vi "GPIB write expt GPIB.vi"(0 "Command list 1":T1(array[cluster]) {"Module" items=["TTL high                                                                                 ", "TTL low                          ", "Camera Strobe                   ", "CMOT", "Defaults                           ", "Fluorescence pulse           ", "IP trap                         ", "Kinetics OD image          ", "Kinetics picture", "Kinetics probe pulse", "MOT light only                ", "MOT off                                   ", "MOT on                         ", "Move cart                      ", "OD image                     ", "Optical pumping          ", "Picture                             ", "Probe Pulse", "Quadrupole trap             ", "IP off", "Utility Module 02           ", "Utility Module 03           ", "Molasses          ", "Utility Module 04     ", "Utility Module 05     ", "Utility Module 06     ", "Utility Module 07     ", "Utility Module 08     ", "Utility Module 09     ", "Utility Module 10     ", "Static DAC", "GPIB"]; "Abs Start Time" format="%.3f"}, 1 "End time":dbl=83073.546, 2 "Abs start time":dbl=62269.999980926514, 3 "do it!":bool=TRUE) -> ()   [LabVIEW 2017]
doc: "This sends out GPIB commands during the experiment (after the DIO (TTL) board has been triggered."
uses:
  globals/Modules global.vi
panel:
  out "Array 2":dbl[](array[numeric])
  out "Array":string[](array[string])
  out "sorted array":T1(array[cluster])
  out "total time":dbl
  out "start time":dbl=3231522488.434
  in  "timeout ms":i32=1000
  out "error out":errorcluster
  # "enabled  time                                      GPIB address                       command"
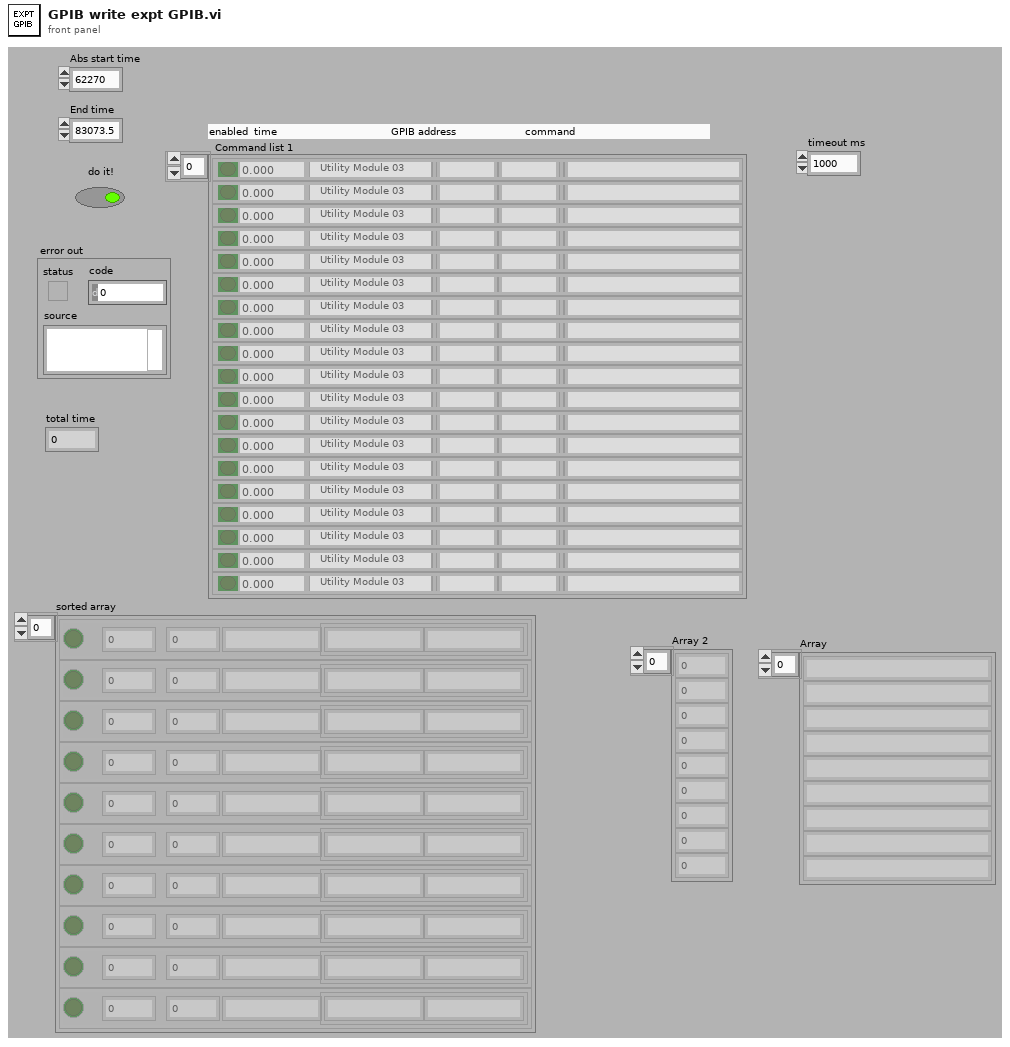
[diagram p1: front panel]
types:
  T1 = cluster{"Enable":bool, "Abs Start Time":dbl, "Module":u16, "String":string, "Array":string[]}[]
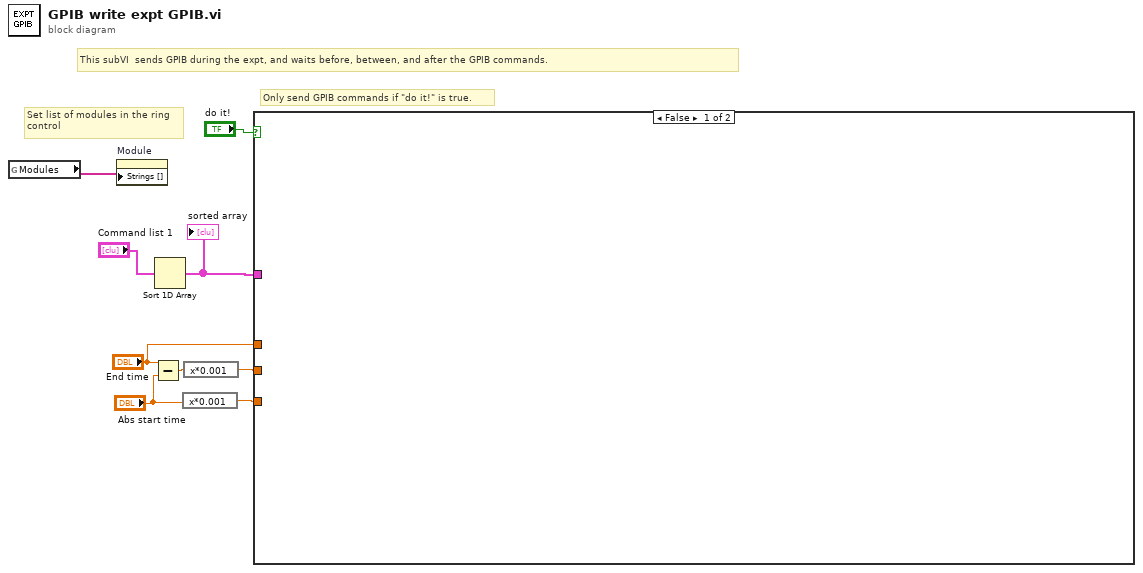
[diagram p0: block diagram]
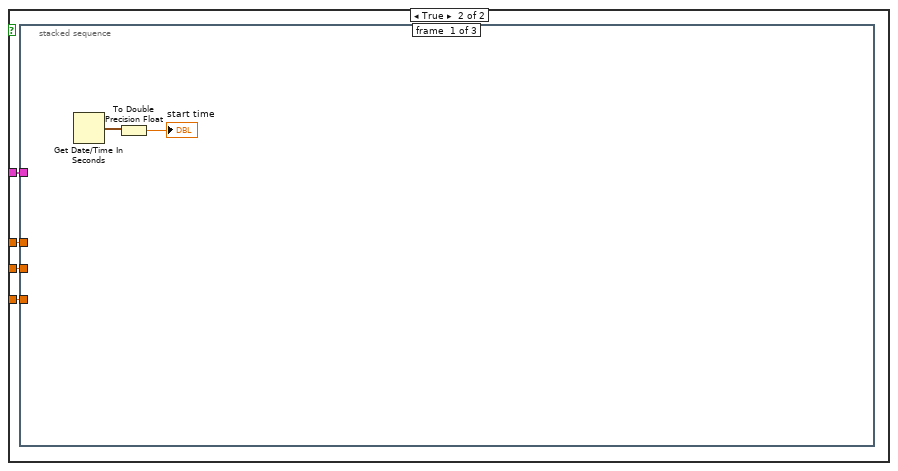
[diagram p2: hidden frame]
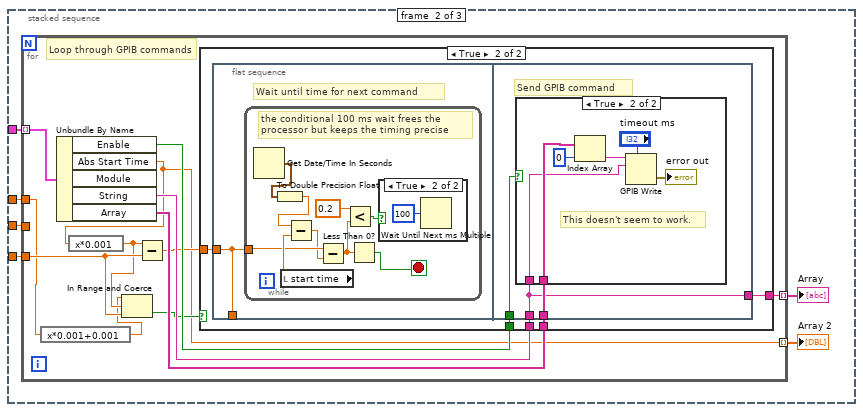
[diagram p3: hidden frame]
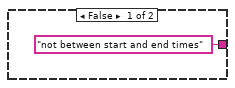
[diagram p4: hidden frame]
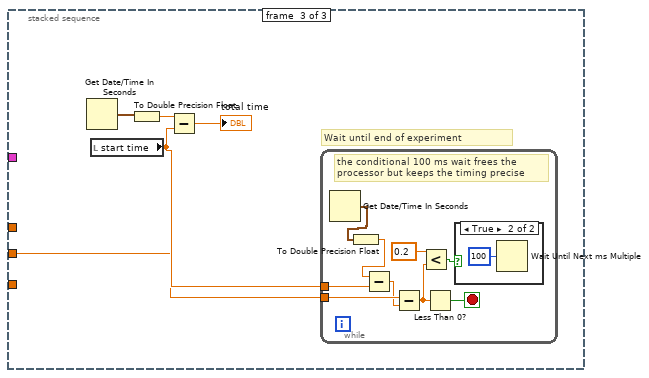
[diagram p7: hidden frame]
diagram:
  # "Set list of modules in the ring control"
  # "Only send GPIB commands if \"do it!\" is true."
  # "This subVI  sends GPIB during the expt, and waits before, between, and after the GPIB commands."
  n1 = global read "Modules global.vi" "Modules"() -> (w1:string[])
  n2 = property on="Module" class="Ring (strict)"("Strings []"=w1) -> ()  [unwired: 2 in, 2 out]
  n3 = Subtract(x="End time", y="Abs start time") -> (x-y=w8:dbl)
  n4 = Sort 1D Array(array="Command list 1") -> (sorted array=w3:T1)
  "sorted array" <- w3
  n5 = expression code="x*0.001"("Abs start time") -> (w5:dbl)
  n6 = expression code="x*0.001"(w8) -> (w7:dbl)
  n7 = case shown="False" "do it!" {
    tunnel: w5 -> [_ w13]
    tunnel: w7 -> [_ w12]
    tunnel: w3 -> [_ w11]
    tunnel: "End time" -> [_ w10]
    frame False {
    }
    frame True {
      n8 = stacked-sequence {
        tunnel: w13 -> [_ w21 _]
        tunnel: w12 -> [_ w18 w60]
        tunnel: w11 -> [_ w20 _]
        tunnel: w10 -> [_ w17 _]
        frame #0 {
          n9 = Get Date/Time In Seconds() -> (seconds since 1Jan1904=w15:timestamp)
          n10 = To Double Precision Float(number=w15) -> (double precision float=→"start time":dbl)
        }
        frame #1 {
          n11 = for {
            tunnel: w20 -> [w33] mode=indexing
            tunnel: w21 -> [w27]
            tunnel: w18 -> [_]
            tunnel: [w26] -> w16 mode=indexing
            tunnel: [w22] -> w19 mode=indexing
            tunnel: w17 -> [w24]
            # "Loop through GPIB commands"
            n12 = expression code="x*0.001+0.001"(w24) -> (w23:dbl)
            n13 = Unbundle By Name(w33) -> ("Enable"=w30:bool, "Abs Start Time"=w22:dbl, "String"=w32:string, "Array"=w31:string[])  [unwired: 1 out]
            n14 = expression code="x*0.001"(w22) -> (w25:dbl)
            n15 = In Range and Coerce(upper limit=w23, x=w25, lower limit=w27) -> (In Range?=w28:bool)  [unwired: 1 out]
            n16 = Subtract(x=w25, y=w27) -> (x-y=w29:dbl)
            n17 = case shown="True" w28 {
              tunnel: w32 -> [_ w39]
              tunnel: w31 -> [_ w38]
              tunnel: w30 -> [_ w37]
              tunnel: w29 -> [_ w36]
              tunnel: ["not between start and end times" ("String") w35] -> w26
              frame False {
              }
              frame True {
                n18 = flat-sequence {
                  tunnel: w36 -> [w40]
                  tunnel: [w40] -> _
                  tunnel: w39 -> [w51]
                  tunnel: w38 -> [w53]
                  tunnel: w37 -> [w52]
                  tunnel: [w51] -> w35
                  frame #0 {
                    # "Wait until time for next command"
                    n19 = while {
                      tunnel: w40 -> [w42]
                      stop <- w46 stop-if-true
                      # "the conditional 100 ms wait frees the processor but keeps the timing precise"
                      n20 = Get Date/Time In Seconds() -> (seconds since 1Jan1904=w45:timestamp)
                      n21 = To Double Precision Float(number=w45) -> (double precision float=w44:dbl)
                      n22 = local read "start time"() -> (w43:dbl)
                      n23 = Subtract(x=w44, y=w43) -> (x-y=w41:dbl)
                      n24 = Subtract(x=w42, y=w41) -> (x-y=w47:dbl)
                      n25 = Less?(x=0.2 ("y"), y=w47) -> (x < y?=w48:bool)
                      n26 = Less Than 0?(x=w47) -> (x < 0?=w46:bool)
                      n27 = case shown="True" w48 {
                        frame False {
                        }
                        frame True {
                          n28 = Wait Until Next ms Multiple(millisecond multiple=u32 100) -> ()  [unwired: 1 out]
                        }
                      }
                    }
                  }
                  frame #1 {
                    # "Send GPIB command"
                    n29 = case shown="True" w52 {
                      tunnel: w51 -> [_ w54]
                      tunnel: w53 -> [_ w55]
                      frame False {
                      }
                      frame True {
                        # "This doesn't seem to work."
                        n30 = Index Array(array=w55, index=0) -> (element=w56:string)
                        n31 = GPIB Write(0:w56, 1:w54, 4:"timeout ms") -> (6:→"error out":errorcluster)  [unwired: 2 in, 1 out]
                      }
                    }
                  }
                }
              }
            }
          }
          "Array" <- w16
          "Array 2" <- w19
        }
        frame #2 {
          # "Wait until end of experiment"
          n32 = Get Date/Time In Seconds() -> (seconds since 1Jan1904=w64:timestamp)
          n33 = local read "start time"() -> (w61:dbl)
          n34 = To Double Precision Float(number=w64) -> (double precision float=w63:dbl)
          n35 = Subtract(x=w63, y=w61) -> (x-y=→"total time":dbl)
          n36 = while {
            tunnel: w61 -> [w67]
            tunnel: w60 -> [w66]
            stop <- w70 stop-if-true
            # "the conditional 100 ms wait frees the processor but keeps the timing precise"
            n37 = Get Date/Time In Seconds() -> (seconds since 1Jan1904=w68:timestamp)
            n38 = To Double Precision Float(number=w68) -> (double precision float=w69:dbl)
            n39 = Subtract(x=w69, y=w67) -> (x-y=w65:dbl)
            n40 = Subtract(x=w66, y=w65) -> (x-y=w71:dbl)
            n41 = Less?(x=0.2 ("y"), y=w71) -> (x < y?=w72:bool)
            n42 = Less Than 0?(x=w71) -> (x < 0?=w70:bool)
            n43 = case shown="True" w72 {
              frame False {
              }
              frame True {
                n44 = Wait Until Next ms Multiple(millisecond multiple=u32 100) -> ()  [unwired: 1 out]
              }
            }
          }
        }
      }
    }
  }
